vi "AlliGator Recompute Decay Statistics Histograms.vi"(7 "Decay Statistics Graph":refnum<vi>, 8 "Error In":errorcluster, 9 "Decay Statistics Bin":i32, 10 "Decays Min Values":sgl[](array[numeric]), 11 "Decays Max Values":sgl[](array[numeric])) -> (0 "Error Out":errorcluster)   [LabVIEW 2021, in "AlliGator Decay Statistics.lvlib"]
doc: "Rebins decay Min & Max histograms."
uses:
  AlliGator Decay Statistics.lvlib
  Graphs/XY Graph/XY Graph Add-Ons.lvlib
  Histograms/Histogram Bin Position.ctl
  Histograms/Histogram Window.lvlib
  Histograms/Linear Histogram Options.ctl
  Histograms/Histogram Bin Option.ctl
  1f021b7e-425b-40a9-9546-7345520a62a8.vi
  b5ad749e-8322-46bf-8c18-040d7131fb1e.vi
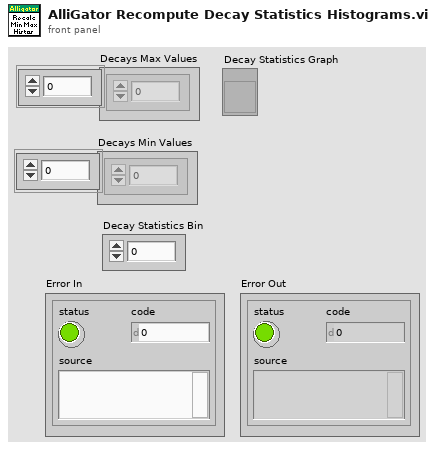
[diagram p1: front panel]
types:
  T1 = typedef "Histogram Window.lvlib/Linear Histogram Options.ctl" = cluster{"Bin Size":dbl, "Bin Number":i32, "Bin Option":T2, "Min Value":dbl, "Max Value":dbl, "Filter NaN & Infinite Values":bool, "Frequency Plot":bool, "Align Bins":bool, "Bin Location":T3, "Project Outside Values":bool, "Max Histogram Size":i32}
  T2 = typedef "Histogram Window.lvlib/Histogram Bin Option.ctl" = enum32{"Bin Number", "Bin Size"}
  T3 = typedef "Histogram Window.lvlib/Histogram Bin Position.ctl" = enum16{"Left", "Center", "Right"}
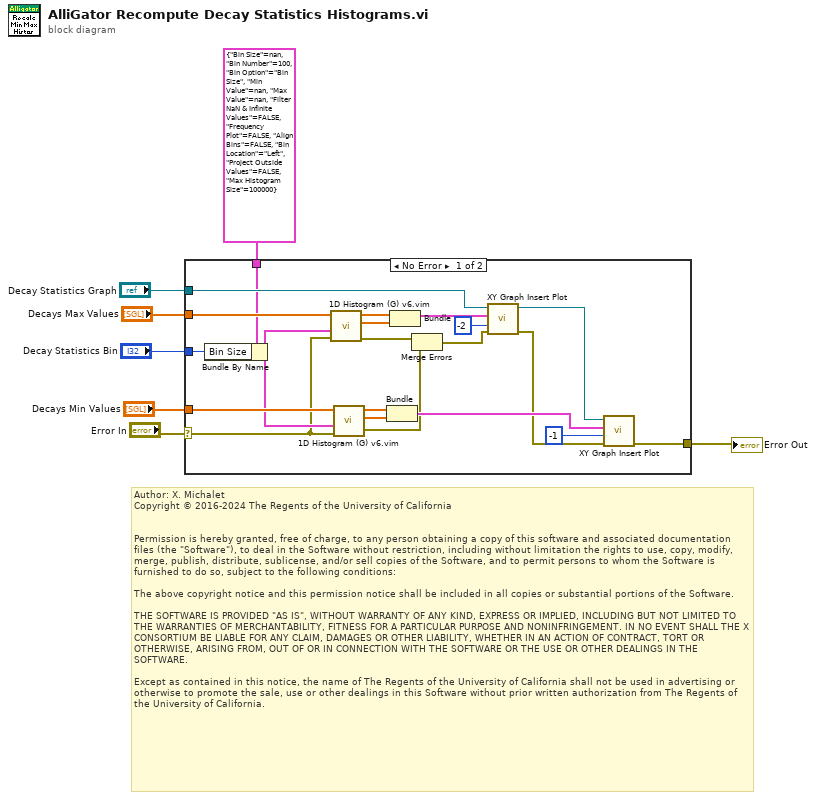
[diagram p0: block diagram]
diagram:
  # "Author: X. Michalet\nCopyright © 2016-2024 The Regents of the University of California\n \n\nPermission is hereby granted, free of charge, to any person obtaining a copy of this software and associated documentation files (the \"Software\"), to deal in the Software without restriction, including without limitation the rights to use, copy, modify, merge, publish, distribute, sublicense, and/or sell copies of the Software, and to permit persons to whom the Software is furnished to do so, subject to the following conditions:\n\nThe above copyright notice and this permission notice shall be included in all copies or substantial portions of the Software.\n\nTHE SOFTWARE IS PROVIDED \"AS IS\", WITHOUT WARRANTY OF ANY KIND, EXPRESS OR IMPLIED, INCLUDING BUT NOT LIMITED TO THE WARRANTIES OF MERCHANTABILITY, FITNESS FOR A PARTICULAR PURPOSE AND NONINFRINGEMENT. IN NO EVENT SHALL THE X CONSORTIUM BE LIABLE FOR ANY CLAIM, DAMAGES OR OTHER LIABILITY, WHETHER IN AN ACTION OF CONTRACT, TORT OR OTHERWISE, ARISING FROM, OUT OF OR IN CONNECTION WITH THE SOFTWARE OR THE USE OR OTHER DEALINGS IN THE SOFTWARE.\n\nExcept as contained in this notice, the name of The Regents of the University of California shall not be used in advertising or otherwise to promote the sale, use or other dealings in this Software without prior written authorization from The Regents of the University of California."
  n1 = case shown="No Error" "Error In" {
    selector: "Error In" -> [w10 w29]
    tunnel: "Decays Max Values" -> [w24 _]
    tunnel: "Decays Min Values" -> [w23 _]
    tunnel: "Decay Statistics Bin" -> [w13 _]
    tunnel: "Decay Statistics Graph" -> [w21 _]
    tunnel: [w15 w29] -> w2
    tunnel: T1 {"Bin Size"=nan, "Bin Number"=100, "Bin Option"=enum."Bin Size", "Min Value"=nan, "Max Value"=nan, "Filter NaN & Infinite Values"=FALSE, "Frequency Plot"=FALSE, "Align Bins"=FALSE, "Bin Location"=enum."Left", "Project Outside Values"=FALSE, "Max Histogram Size"=100000} ("Histogram Options") -> [w14 _]
    frame No Error {
      n2 = Bundle By Name(cluster=w14, "Bin Size"=w13) -> (w12:T1)
      n3 = call "1D Histogram (G) v6.vim"("Error In"=w10, "Histogram Options"=w12, "Array"=w24) -> ("Error Out"=w11:errorcluster, "Histogram"=w27:dbl[], "Axis"=w28:dbl[])  [unwired: 2 in, 4 out]
      n4 = call "1D Histogram (G) v6.vim"("Error In"=w10, "Histogram Options"=w12, "Array"=w23) -> ("Error Out"=w8:errorcluster, "Histogram"=w25:dbl[], "Axis"=w26:dbl[])  [unwired: 2 in, 4 out]
      n5 = Bundle("Axis"=w26, "Histogram"=w25) -> (w19:cluster{"Axis":dbl[], "Histogram":dbl[]})  [unwired: 1 in]
      n6 = Bundle("Axis"=w28, "Histogram"=w27) -> (w22:cluster{"Axis":dbl[], "Histogram":dbl[]})  [unwired: 1 in]
      n7 = Merge Errors(w11, w8) -> (w9:errorcluster)
      n8 = call "XY Graph Insert Plot.vi"("Error In"=w9, "Plot Index (Default Inf: Append to End)"=-2, "New Plot"=w22, "Multiplot XY Graph Refnum in"=w21) -> ("Error Out"=w17:errorcluster, "Multiplot XY Graph Refnum out"=w18:refnum<vi>)  [unwired: 5 in, 1 out]
      n9 = call "XY Graph Insert Plot.vi"("Error In"=w17, "Plot Index (Default Inf: Append to End)"=-1, "New Plot"=w19, "Multiplot XY Graph Refnum in"=w18) -> ("Error Out"=w15:errorcluster)  [unwired: 5 in, 2 out]
    }
    frame Error {
    }
  }
  "Error Out" <- w2
